vi "Catch_screw(show_side).vi"(6 "向哪校正":T1(ring)=enum."left", 7 "櫃子在哪?":enum16{"前面", "左邊", "右邊"}(ring), 8 "Error In":errorcluster) -> (0 "Error Out":errorcluster, 3 "it2(nut)":string)   [LabVIEW 2019]
uses:
  WSCbot_V3_Toolkit.lvlibp/WSCBOTV3_Toolkit/IO/LowLevel/PulseCounter.ctl
  WSCbot_V3_Toolkit.lvlibp
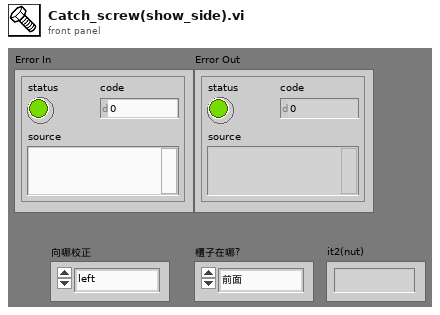
[diagram p1: front panel]
types:
  T1 = enum16{"Right_up", "Right_down", "Left_down", "Left_up", "left", "right", "up", "down"}
  T2 = typedef "WSCbot_V3_Toolkit.lvlibp/PulseCounter.ctl" = enum16{"CH1", "CH2", "CH3", "CH4", "CH5"}
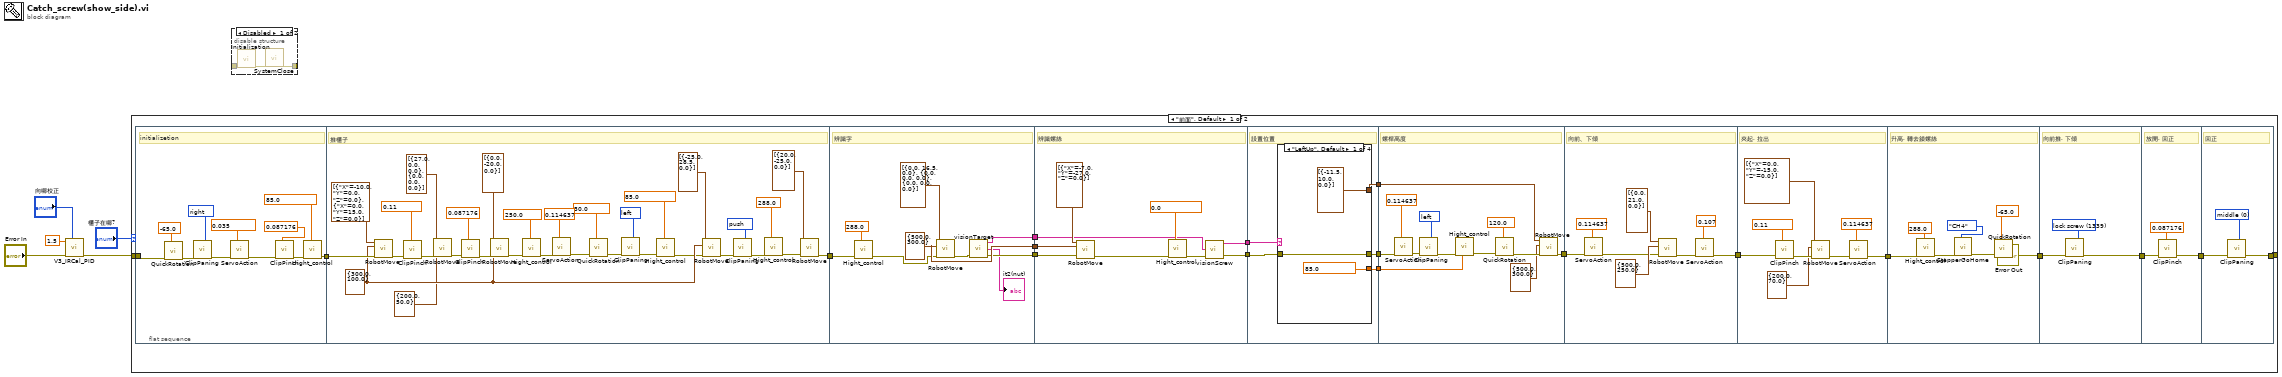
[diagram p0: block diagram]
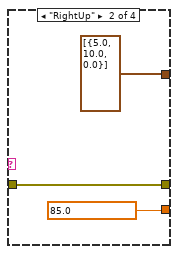
[diagram p2: hidden frame]
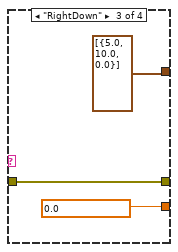
[diagram p3: hidden frame]
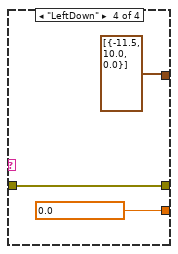
[diagram p4: hidden frame]
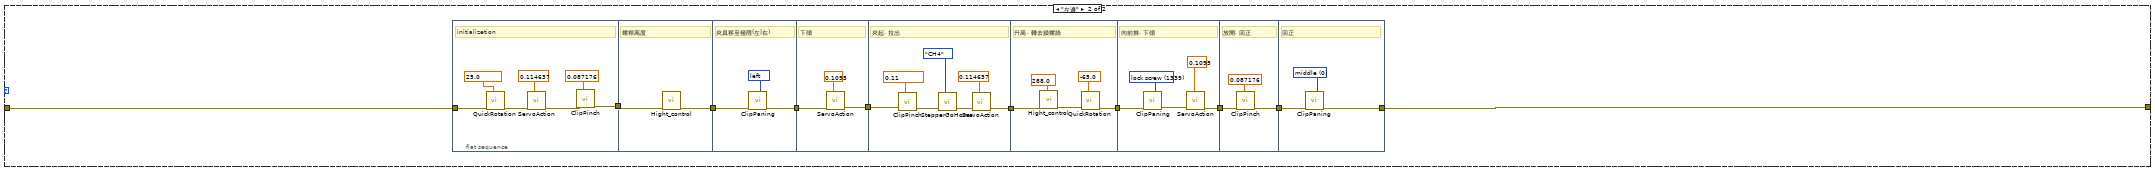
[diagram p5: hidden frame]
diagram:
  n1 = call "V3_IRCal_PID.vi"("Direction"="向哪校正", "Error In"="Error In", "X_distance(V)"=1.5) -> ("Error Out"=w4:errorcluster)  [unwired: 7 in, 1 out]
  n2 = case shown="\"前面\", Default" "櫃子在哪?" {
    tunnel: [w18 w147] -> w6
    tunnel: w4 -> [w19 w146]
    frame "前面", Default {
      n3 = flat-sequence {
        tunnel: w19 -> [w34]
        tunnel: [w27] -> w7
        tunnel: [w43] -> w8
        tunnel: w7 -> [w61]
        tunnel: w8 -> [w69]
        tunnel: [w74] -> w17
        tunnel: [w73] -> w16
        tunnel: [w71] -> w15
        tunnel: w17 -> [w78]
        tunnel: w16 -> [w82]
        tunnel: w15 -> [w81]
        tunnel: [w77] -> w13
        tunnel: [w79] -> w12
        tunnel: w13 -> [w89]
        tunnel: w12 -> [w88]
        tunnel: [w87] -> w11
        tunnel: [w86] -> w10
        tunnel: [w85] -> w9
        tunnel: [w112] -> w14
        tunnel: w11 -> [w111]
        tunnel: w10 -> [w109]
        tunnel: w9 -> [w106]
        tunnel: [w121] -> w24
        tunnel: w14 -> [w116]
        tunnel: [w127] -> w23
        tunnel: w24 -> [w128]
        tunnel: w23 -> [w135]
        tunnel: [w136] -> w22
        tunnel: w22 -> [w139]
        tunnel: [w137] -> w21
        tunnel: w21 -> [w142]
        tunnel: [w140] -> w20
        tunnel: w20 -> [w144]
        tunnel: [w143] -> w18
        frame #0 {
          w25 = -65.0 items=["Forward"=30.0, "Right"=120.0, "Left"=-65.0] ("螺桿面向")
          w26 = 85.0 items=["物料櫃第一格"=0.0, "物料櫃第二格"=85.0, "螺帽夾取高度"=128.0, "螺帽瞄準"=250.0, "最高"=288.0] ("螺桿高度")
          w29 = -3500 items=["left"=2300, "right"=-3500, "lock screw"=1345, "lock_nut"=1167, "middle"=0] ("location")
          w33 = 0.035 items=["up"=0.1095, "lock_up"=0.111528, "up_up"=0.114637, "down"=0.073446, "back"=0.037435, "back_back"=0.035] ("face_dir")
          w35 = 0.087176 items=["pinch_up"=0.11, "release"=0.087176] ("pinch?")
          # "initializetion"
          n4 = call "QuickRotation.vi"("螺桿面向"=w25, "Error In"=w34) -> ("Error Out"=w31:errorcluster)  [unwired: 9 in]
          n5 = call "ClipPaning.vi"("Error In"=w31, "location"=w29) -> ("Error Out"=w30:errorcluster)  [unwired: 8 in]
          n6 = call "ServoAction.vi"("face_dir"=w33, "Error In"=w30) -> ("Error Out"=w32:errorcluster)  [unwired: 9 in]
          n7 = call "ClipPinch.vi"("pinch?"=w35, "Error In"=w32) -> ("Error Out"=w28:errorcluster)  [unwired: 9 in]
          n8 = call "Hight_control.vi"("螺桿高度"=w26, "Error In"=w28) -> ("Error Out"=w27:errorcluster)  [unwired: 9 in]
        }
        frame #1 {
          w36 = -1800 items=["left"=2250, "right"=-3500, "lock screw"=1345, "lock_nut"=1167, "push"=-1800, "middle"=0] ("location")
          w38 = 30.0 items=["Forward"=30.0, "Right"=120.0, "Left"=-65.0] ("螺桿面向")
          w39 = 288.0 items=["物料櫃第一格"=0.0, "物料櫃第二格"=85.0, "螺帽夾取高度"=128.0, "螺帽瞄準"=250.0, "最高"=288.0] ("螺桿高度")
          w44 = 85.0 items=["物料櫃第一格"=0.0, "物料櫃第二格"=85.0, "螺帽夾取高度"=128.0, "螺帽瞄準"=250.0, "最高"=288.0] ("螺桿高度")
          w47 = 2250 items=["left"=2250, "right"=-3500, "lock screw"=1345, "lock_nut"=1167, "middle"=0] ("location")
          w49 = 250.0 items=["物料櫃第一格"=0.0, "物料櫃第二格"=85.0, "螺帽夾取高度"=128.0, "螺帽瞄準"=250.0, "最高"=288.0] ("螺桿高度")
          w55 = 0.114637 items=["up"=0.1095, "lock_up"=0.111528, "up_up"=0.114637, "down"=0.073446, "back"=0.037435, "back_back"=0.035] ("face_dir")
          w57 = 0.087176 items=["pinch_up"=0.11, "release"=0.087176] ("pinch?")
          w64 = 0.11 items=["pinch_up"=0.11, "release"=0.087176] ("pinch?")
          w53 = cluster{dbl, dbl} {300.0, 100.0} ("Speed/ACC")
          # "推櫃子"
          n9 = call "RobotMove.vi"("error in (no error)"=w61, "Speed/ACC"=w53, "XYZ"=cluster{"X":dbl, "Y":dbl, "Z":dbl}[] [{"X"=-10.0, "Y"=0.0, "Z"=0.0}, {"X"=0.0, "Y"=15.0, "Z"=0.0}]) -> ("error out"=w65:errorcluster)  [unwired: 8 in]
          n10 = call "ClipPinch.vi"("pinch?"=w64, "Error In"=w65) -> ("Error Out"=w63:errorcluster)  [unwired: 9 in]
          n11 = call "RobotMove.vi"("error in (no error)"=w63, "Speed/ACC"=cluster{dbl, dbl} {200.0, 50.0}, "XYZ"=cluster{"X":dbl, "Y":dbl, "Z":dbl}[] [{"X"=27.0, "Y"=0.0, "Z"=0.0}, {"X"=0.0, "Y"=0.0, "Z"=0.0}]) -> ("error out"=w59:errorcluster)  [unwired: 8 in]
          n12 = call "ClipPinch.vi"("pinch?"=w57, "Error In"=w59) -> ("Error Out"=w58:errorcluster)  [unwired: 9 in]
          n13 = call "RobotMove.vi"("error in (no error)"=w58, "Speed/ACC"=w53, "XYZ"=cluster{"X":dbl, "Y":dbl, "Z":dbl}[] [{"X"=0.0, "Y"=-20.0, "Z"=0.0}]) -> ("error out"=w51:errorcluster)  [unwired: 8 in]
          n14 = call "Hight_control.vi"("螺桿高度"=w49, "Error In"=w51) -> ("Error Out"=w50:errorcluster)  [unwired: 9 in]
          n15 = call "ServoAction.vi"("face_dir"=w55, "Error In"=w50) -> ("Error Out"=w56:errorcluster)  [unwired: 9 in]
          n16 = call "QuickRotation.vi"("螺桿面向"=w38, "Error In"=w56) -> ("Error Out"=w48:errorcluster)  [unwired: 9 in]
          n17 = call "ClipPaning.vi"("Error In"=w48, "location"=w47) -> ("Error Out"=w46:errorcluster)  [unwired: 8 in]
          n18 = call "Hight_control.vi"("螺桿高度"=w44, "Error In"=w46) -> ("Error Out"=w45:errorcluster)  [unwired: 9 in]
          n19 = call "RobotMove.vi"("error in (no error)"=w45, "Speed/ACC"=w53, "XYZ"=cluster{"X":dbl, "Y":dbl, "Z":dbl}[] [{"X"=-25.0, "Y"=28.5, "Z"=0.0}]) -> ("error out"=w54:errorcluster)  [unwired: 8 in]
          n20 = call "ClipPaning.vi"("Error In"=w54, "location"=w36) -> ("Error Out"=w41:errorcluster)  [unwired: 8 in]
          n21 = call "Hight_control.vi"("螺桿高度"=w39, "Error In"=w41) -> ("Error Out"=w40:errorcluster)  [unwired: 9 in]
          n22 = call "RobotMove.vi"("error in (no error)"=w40, "XYZ"=cluster{"X":dbl, "Y":dbl, "Z":dbl}[] [{"X"=20.0, "Y"=-25.0, "Z"=0.0}]) -> ("error out"=w43:errorcluster)  [unwired: 9 in]
        }
        frame #2 {
          w68 = 288.0 items=["物料櫃第一格"=0.0, "物料櫃第二格"=85.0, "螺帽夾取高度"=128.0, "螺帽瞄準"=250.0, "最高"=288.0] ("螺桿高度")
          w73 = cluster{dbl, dbl} {500.0, 300.0} ("Speed/ACC")
          # "辨識字"
          n23 = call "Hight_control.vi"("螺桿高度"=w68, "Error In"=w69) -> ("Error Out"=w67:errorcluster)  [unwired: 9 in]
          n24 = call "RobotMove.vi"("error in (no error)"=w67, "Speed/ACC"=w73, "XYZ"=cluster{"X":dbl, "Y":dbl, "Z":dbl}[] [{"X"=0.0, "Y"=16.5, "Z"=0.0}, {"X"=0.0, "Y"=0.0, "Z"=0.0}, {"X"=0.0, "Y"=0.0, "Z"=0.0}]) -> ("error out"=w72:errorcluster)  [unwired: 8 in]
          n25 = call "visionTarget.vi"("Error In"=w72) -> ("Error Out"=w71:errorcluster, "it2(nut)"=→"it2(nut)":string, "it1(screw)"=w74:string)  [unwired: 2 in]
        }
        frame #3 {
          w83 = 0.0 items=["物料櫃第一格"=0.0, "物料櫃第二格"=78.0, "螺帽夾取高度"=128.0, "螺帽瞄準"=250.0, "最高"=288.0] ("螺桿高度")
          # "辨識螺絲"
          n26 = call "RobotMove.vi"("error in (no error)"=w81, "Speed/ACC"=w82, "XYZ"=cluster{"X":dbl, "Y":dbl, "Z":dbl}[] [{"X"=-7.0, "Y"=-27.0, "Z"=0.0}]) -> ("error out"=w76:errorcluster)  [unwired: 8 in]
          n27 = call "Hight_control.vi"("螺桿高度"=w83, "Error In"=w76) -> ("Error Out"=w80:errorcluster)  [unwired: 9 in]
          n28 = call "visionScrew.vi"("Error In"=w80, "Aim_Color"=w78) -> ("Error Out"=w79:errorcluster, "Position"=w77:string)  [unwired: 2 in]
        }
        frame #4 {
          # "設置位置"
          n29 = case shown="\"LeftUp\", Default" w89 {
            tunnel: [w90 w93 w98 w99] -> w85
            tunnel: w88 -> [w91 w94 w96 w100]
            tunnel: [cluster{"X":dbl, "Y":dbl, "Z":dbl}[] [{"X"=-11.5, "Y"=10.0, "Z"=0.0}] ("XYZ") cluster{"X":dbl, "Y":dbl, "Z":dbl}[] [{"X"=5.0, "Y"=10.0, "Z"=0.0}] ("XYZ") cluster{"X":dbl, "Y":dbl, "Z":dbl}[] [{"X"=5.0, "Y"=10.0, "Z"=0.0}] ("XYZ") cluster{"X":dbl, "Y":dbl, "Z":dbl}[] [{"X"=-11.5, "Y"=10.0, "Z"=0.0}] ("XYZ")] -> w87
            tunnel: [w91 w94 w96 w100] -> w86
            frame "LeftUp", Default {
              w90 = 85.0 items=["物料櫃第一格"=0.0, "物料櫃第二格"=85.0, "螺帽夾取高度"=128.0, "螺帽瞄準"=250.0, "最高"=288.0] ("螺桿高度")
            }
            frame "RightUp" {
              w93 = 85.0 items=["物料櫃第一格"=0.0, "物料櫃第二格"=85.0, "螺帽夾取高度"=128.0, "螺帽瞄準"=250.0, "最高"=288.0] ("螺桿高度")
            }
            frame "RightDown" {
              w98 = 0.0 items=["物料櫃第一格"=0.0, "物料櫃第二格"=78.0, "螺帽夾取高度"=128.0, "螺帽瞄準"=250.0, "最高"=288.0] ("螺桿高度")
            }
            frame "LeftDown" {
              w99 = 0.0 items=["物料櫃第一格"=0.0, "物料櫃第二格"=78.0, "螺帽夾取高度"=128.0, "螺帽瞄準"=250.0, "最高"=288.0] ("螺桿高度")
            }
          }
        }
        frame #5 {
          w102 = 120.0 items=["Forward"=30.0, "Right"=120.0, "Left"=-65.0] ("螺桿面向")
          w103 = 2300 items=["left"=2300, "right"=-3500, "lock screw"=1345, "lock_nut"=1167, "middle"=0] ("location")
          w107 = 0.114637 items=["up"=0.1095, "lock_up"=0.111528, "up_up"=0.114637, "down"=0.073446, "back"=0.037435, "back_back"=0.035] ("face_dir")
          # "螺桿高度"
          n30 = call "ServoAction.vi"("face_dir"=w107, "Error In"=w109) -> ("Error Out"=w108:errorcluster)  [unwired: 9 in]
          n31 = call "ClipPaning.vi"("Error In"=w108, "location"=w103) -> ("Error Out"=w105:errorcluster)  [unwired: 8 in]
          n32 = call "Hight_control.vi"("螺桿高度"=w106, "Error In"=w105) -> ("Error Out"=w104:errorcluster)  [unwired: 9 in]
          n33 = call "QuickRotation.vi"("螺桿面向"=w102, "Error In"=w104) -> ("Error Out"=w113:errorcluster)  [unwired: 9 in]
          n34 = call "RobotMove.vi"("error in (no error)"=w113, "Speed/ACC"=cluster{dbl, dbl} {500.0, 300.0}, "XYZ"=w111) -> ("error out"=w112:errorcluster)  [unwired: 8 in]
        }
        frame #6 {
          w114 = 0.107 items=["up"=0.107, "lock_up"=0.111528, "up_up"=0.114637, "down"=0.073446, "back"=0.037435, "back_back"=0.035] ("face_dir")
          w117 = 0.114637 items=["up"=0.1095, "up_up"=0.114637, "down"=0.073446, "back"=0.037435, "back_back"=0.035] ("face_dir")
          # "向前、下傾"
          n35 = call "ServoAction.vi"("face_dir"=w117, "Error In"=w116) -> ("Error Out"=w115:errorcluster)  [unwired: 9 in]
          n36 = call "RobotMove.vi"("error in (no error)"=w115, "Speed/ACC"=cluster{dbl, dbl} {500.0, 250.0}, "XYZ"=cluster{"X":dbl, "Y":dbl, "Z":dbl}[] [{"X"=0.0, "Y"=21.0, "Z"=0.0}]) -> ("error out"=w120:errorcluster)  [unwired: 8 in]
          n37 = call "ServoAction.vi"("face_dir"=w114, "Error In"=w120) -> ("Error Out"=w121:errorcluster)  [unwired: 9 in]
        }
        frame #7 {
          w126 = 0.114637 items=["up"=0.1095, "up_up"=0.114637, "down"=0.073446, "back"=0.037435, "back_back"=0.035] ("face_dir")
          w129 = 0.11 items=["pinch_up"=0.11, "release"=0.087176] ("pinch?")
          # "夾起, 拉出"
          n38 = call "ClipPinch.vi"("pinch?"=w129, "Error In"=w128) -> ("Error Out"=w125:errorcluster)  [unwired: 9 in]
          n39 = call "RobotMove.vi"("error in (no error)"=w125, "Speed/ACC"=cluster{dbl, dbl} {200.0, 70.0}, "XYZ"=cluster{"X":dbl, "Y":dbl, "Z":dbl}[] [{"X"=0.0, "Y"=-15.0, "Z"=0.0}]) -> ("error out"=w124:errorcluster)  [unwired: 8 in]
          n40 = call "ServoAction.vi"("face_dir"=w126, "Error In"=w124) -> ("Error Out"=w127:errorcluster)  [unwired: 9 in]
        }
        frame #8 {
          w130 = -65.0 items=["Forward"=30.0, "Right"=120.0, "Left"=-65.0] ("螺桿面向")
          w134 = 288.0 items=["物料櫃第一格"=0.0, "物料櫃第二格"=78.0, "螺帽夾取高度"=128.0, "螺帽瞄準"=250.0, "最高"=288.0] ("螺桿高度")
          # "升高, 轉去鎖螺絲"
          n41 = call "Hight_control.vi"("螺桿高度"=w134, "Error In"=w135) -> ("Error Out"=w132:errorcluster)  [unwired: 9 in]
          n42 = call "StepperGoHome.vi"("PulseCounterChanel"=PulseCounter."CH4", "Error In"=w132) -> ("Error Out"=w131:errorcluster)  [unwired: 7 in, 2 out]
          n43 = call "QuickRotation.vi"("螺桿面向"=w130, "Error In"=w131) -> ("Error Out"=w136:errorcluster)  [unwired: 9 in]
        }
        frame #9 {
          w138 = 1339 items=["left"=2100, "right"=-3500, "lock screw"=1339, "middle"=0] ("location")
          # "向前推, 下傾"
          n44 = call "ClipPaning.vi"("Error In"=w139, "location"=w138) -> ("Error Out"=w137:errorcluster)  [unwired: 8 in]
        }
        frame #10 {
          w141 = 0.087176 items=["pinch_up"=0.11, "release"=0.087176] ("pinch?")
          # "放開, 回正"
          n45 = call "ClipPinch.vi"("pinch?"=w141, "Error In"=w142) -> ("Error Out"=w140:errorcluster)  [unwired: 9 in]
        }
        frame #11 {
          w145 = 0 items=["left"=2100, "right"=-3500, "lock screw"=1339, "middle"=0] ("location")
          # "回正"
          n46 = call "ClipPaning.vi"("Error In"=w144, "location"=w145) -> ("Error Out"=w143:errorcluster)  [unwired: 8 in]
        }
      }
    }
    frame "左邊" {
      n47 = flat-sequence {
        tunnel: [w159] -> w155
        tunnel: w146 -> [w157]
        tunnel: w155 -> [w164]
        tunnel: [w163] -> w154
        tunnel: [w167] -> w153
        tunnel: w154 -> [w165]
        tunnel: w153 -> [w169]
        tunnel: [w170] -> w152
        tunnel: [w172] -> w151
        tunnel: w152 -> [w174]
        tunnel: w151 -> [w180]
        tunnel: [w181] -> w150
        tunnel: w150 -> [w187]
        tunnel: [w183] -> w149
        tunnel: w149 -> [w190]
        tunnel: [w188] -> w148
        tunnel: w148 -> [w192]
        tunnel: [w191] -> w147
        frame #0 {
          w156 = 25.0 items=["Forward"=25.0, "Right"=115.0, "Left"=-65.0] ("螺桿面向")
          w161 = 0.087176 items=["pinch_up"=0.11, "release"=0.087176] ("pinch?")
          w162 = 0.114637 items=["up"=0.1095, "up_up"=0.114637, "down"=0.073446, "back"=0.037435, "back_back"=0.035] ("face_dir")
          # "initializetion"
          n48 = call "QuickRotation.vi"("螺桿面向"=w156, "Error In"=w157) -> ("Error Out"=w158:errorcluster)  [unwired: 9 in]
          n49 = call "ServoAction.vi"("face_dir"=w162, "Error In"=w158) -> ("Error Out"=w160:errorcluster)  [unwired: 9 in]
          n50 = call "ClipPinch.vi"("pinch?"=w161, "Error In"=w160) -> ("Error Out"=w159:errorcluster)  [unwired: 9 in]
        }
        frame #1 {
          # "螺桿高度"
          n51 = call "Hight_control.vi"("Error In"=w164) -> ("Error Out"=w163:errorcluster)  [unwired: 10 in]
        }
        frame #2 {
          w166 = 2100 items=["left"=2100, "right"=-3500, "lock screw"=1339, "middle"=0] ("location")
          # "夾具移至極限(左|右)"
          n52 = call "ClipPaning.vi"("Error In"=w165, "location"=w166) -> ("Error Out"=w167:errorcluster)  [unwired: 8 in]
        }
        frame #3 {
          w168 = 0.1095 items=["up"=0.1095, "up_up"=0.114637, "down"=0.073446, "back"=0.037435, "back_back"=0.035] ("face_dir")
          # "下傾"
          n53 = call "ServoAction.vi"("face_dir"=w168, "Error In"=w169) -> ("Error Out"=w170:errorcluster)  [unwired: 9 in]
        }
        frame #4 {
          w171 = 0.114637 items=["up"=0.1095, "up_up"=0.114637, "down"=0.073446, "back"=0.037435, "back_back"=0.035] ("face_dir")
          w177 = 0.11 items=["pinch_up"=0.11, "release"=0.087176] ("pinch?")
          # "夾起, 拉出"
          n54 = call "ClipPinch.vi"("pinch?"=w177, "Error In"=w174) -> ("Error Out"=w176:errorcluster)  [unwired: 9 in]
          n55 = call "StepperGoHome.vi"("PulseCounterChanel"=PulseCounter."CH4", "Error In"=w176) -> ("Error Out"=w173:errorcluster)  [unwired: 7 in, 2 out]
          n56 = call "ServoAction.vi"("face_dir"=w171, "Error In"=w173) -> ("Error Out"=w172:errorcluster)  [unwired: 9 in]
        }
        frame #5 {
          w178 = 288.0 items=["物料櫃第一格"=0.0, "物料櫃第二格"=78.0, "螺帽夾取高度"=128.0, "螺帽瞄準"=250.0, "最高"=288.0] ("螺桿高度")
          w182 = -65.0 items=["Forward"=25.0, "Right"=115.0, "Left"=-65.0] ("螺桿面向")
          # "升高, 轉去鎖螺絲"
          n57 = call "Hight_control.vi"("螺桿高度"=w178, "Error In"=w180) -> ("Error Out"=w179:errorcluster)  [unwired: 9 in]
          n58 = call "QuickRotation.vi"("螺桿面向"=w182, "Error In"=w179) -> ("Error Out"=w181:errorcluster)  [unwired: 9 in]
        }
        frame #6 {
          w184 = 0.1095 items=["up"=0.1095, "up_up"=0.114637, "down"=0.073446, "back"=0.037435, "back_back"=0.035] ("face_dir")
          w186 = 1339 items=["left"=2100, "right"=-3500, "lock screw"=1339, "middle"=0] ("location")
          # "向前推, 下傾"
          n59 = call "ClipPaning.vi"("Error In"=w187, "location"=w186) -> ("Error Out"=w185:errorcluster)  [unwired: 8 in]
          n60 = call "ServoAction.vi"("face_dir"=w184, "Error In"=w185) -> ("Error Out"=w183:errorcluster)  [unwired: 9 in]
        }
        frame #7 {
          w189 = 0.087176 items=["pinch_up"=0.11, "release"=0.087176] ("pinch?")
          # "放開, 回正"
          n61 = call "ClipPinch.vi"("pinch?"=w189, "Error In"=w190) -> ("Error Out"=w188:errorcluster)  [unwired: 9 in]
        }
        frame #8 {
          w193 = 0 items=["left"=2100, "right"=-3500, "lock screw"=1339, "middle"=0] ("location")
          # "回正"
          n62 = call "ClipPaning.vi"("Error In"=w192, "location"=w193) -> ("Error Out"=w191:errorcluster)  [unwired: 8 in]
        }
      }
    }
  }
  "Error Out" <- w6
  n63 = disable-structure shown="Disabled" {
    disable-tunnel: [w195 _] -> _
    disable-tunnel: _ -> [w194 _]
    frame Disabled {
      n64 = call "Initialization.vi"("Error In"=w194) -> ("Error Out"=w195:errorcluster)  [unwired: 10 in]
      n65 = call "SystemClose.vi"() -> ()  [unwired: 3 in, 1 out]
    }
    frame Enabled {
    }
  }
